vi "Actor Test Harness.vi"() -> ()   [LabVIEW 2015]
uses:
  Simple Actor/Simple Actor/Simple Actor.lvclass
  <vilib>/ActorFramework/Actor/Actor.lvclass
panel:
  in  "Update":bool
  in  "Zero Button":bool
  in  "Stop":bool
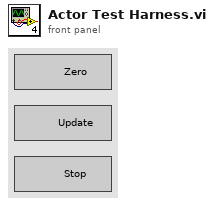
[diagram p1: front panel]
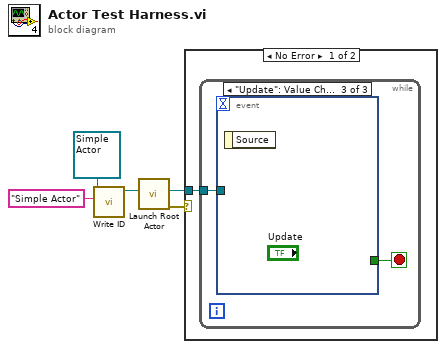
[diagram p0: block diagram]
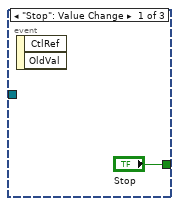
[diagram p2: hidden frame]
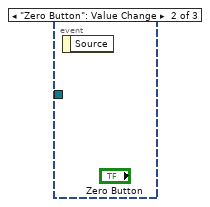
[diagram p3: hidden frame]
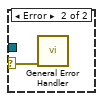
[diagram p4: hidden frame]
diagram:
  n1 = call "Write ID.vi"("ID"="Simple Actor", "Simple Actor in"=refnum<class "Simple Actor.lvclass"> refnum ("Simple Actor.lvlib:Simple Actor.lvclass")) -> ("Simple Actor out"=w3:refnum<class "Simple Actor.lvclass">)  [unwired: 9 in]
  n2 = call <vilib>:"Launch Root Actor.vi"("Actor"=w3) -> ("error out"=w1:errorcluster, "Actor's Enqueuer"=w2:refnum<class "Message Enqueuer.lvclass">)  [unwired: 9 in]
  n3 = case shown="No Error" w1 {
    selector: w1 -> [_ w10]
    tunnel: w2 -> [w6 _]
    frame No Error {
      n4 = while {
        tunnel: w6 -> [w8]
        stop <- w7 stop-if-true
        n5 = event shown="[2] \"Update\": Value Change" {
          selector: _ -> [_ _ _]
          dyn-events: _ -> [_ _ _]
          timeout: _ -> [_ _ _]
          tunnel: w8 -> [_ _ _]
          tunnel: ["Stop" _ _] -> w7
          event "Stop": Value Change {
            n6 = event-data() -> ()  [unwired: 1 in, 2 out]
          }
          event "Zero Button": Value Change {
            n7 = event-data() -> ()  [unwired: 1 in, 1 out]
          }
          event "Update": Value Change {
            n8 = event-data() -> ()  [unwired: 1 in, 1 out]
          }
        }
      }
    }
    frame Error {
      n9 = call <vilib>:"General Error Handler.vi"("error in (no error)"=w10) -> ()  [unwired: 10 in, 5 out]
    }
  }
